vi "Channel_On-Off.vi"(1 "Vertical coupling":dbl, 2 "Enable":bool, 3 "wfm":i8[](array[numeric]), 4 "actual record length":i32) -> (0 "String":string)   [LabVIEW 2011]
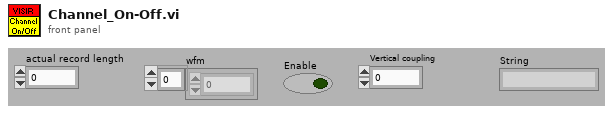
[diagram p1: front panel]
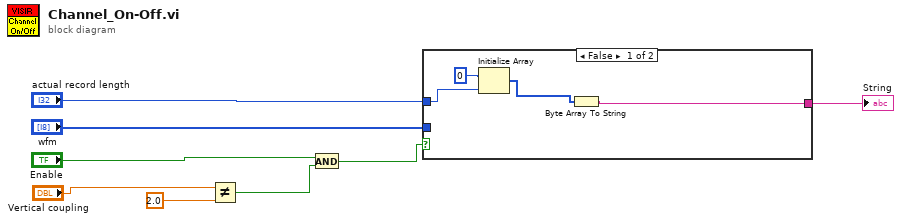
[diagram p0: block diagram]
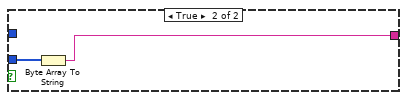
[diagram p2: hidden frame]
diagram:
  n1 = Not Equal?(x="Vertical coupling", y=2.0) -> (x != y?=w6:bool)
  n2 = And(x="Enable", y=w6) -> (x .and. y?=w7:bool)
  n3 = case shown="False" w7 {
    tunnel: "wfm" -> [_ w14]
    tunnel: "actual record length" -> [w11 _]
    tunnel: [w9 w13] -> w4
    frame False {
      n4 = Initialize Array(i8 0 ("element"), w11) -> (w10:i8[])
      n5 = Byte Array To String(unsigned byte array=w10) -> (string=w9:string)
    }
    frame True {
      n6 = Byte Array To String(unsigned byte array=w14) -> (string=w13:string)
    }
  }
  "String" <- w4
